vi "Socket.UDP Multicast Server.vi"() -> ()   [LabVIEW 2014]
uses:
  Classes/Socket.UDP/Socket.UDP.lvclass
  Classes/Socket.UDP/Socket.UDP.lvclass/Socket.UDP.ctl
  Classes/Socket.UDP/Accessors/Write time-to-live.vi
  Classes/Socket.UDP/Accessors/Write transfer_mode.vi
panel:
  out "error out":errorcluster
  in  "Stop Button":bool
  out "Transmitted Strings":string
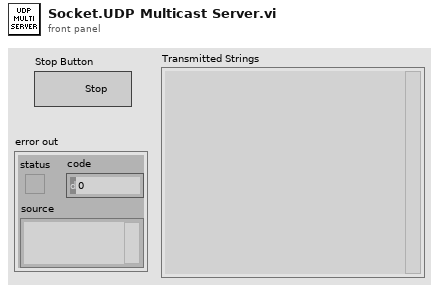
[diagram p1: front panel]
types:
  T1 = enum16{"point-to-point", "multicast", "broadcast"}
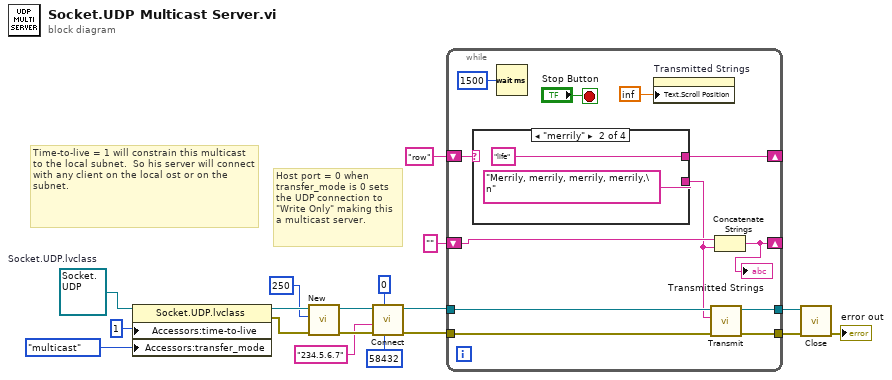
[diagram p0: block diagram]
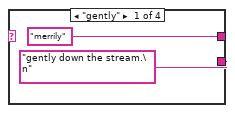
[diagram p2: hidden frame]
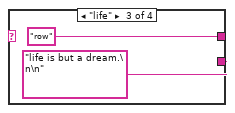
[diagram p3: hidden frame]
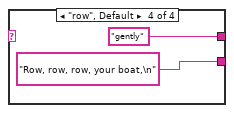
[diagram p4: hidden frame]
diagram:
  w18 = refnum<class "Socket.UDP.lvclass"> refnum  # Socket.UDP.lvclass
  # "Host port = 0 when transfer_mode is 0 sets  the UDP connection to \"Write Only\" making this a multicast server."
  # "Time-to-live = 1 will constrain this multicast to the local subnet.  So his server will connect with any client on the local ost or on the subnet."
  n1 = property class="Socket.UDP.lvclass"(reference=w18, "Accessors:time-to-live"=u16 1 ("time-to-live"), "Accessors:transfer_mode"=T1."multicast" ("transfer_mode")) -> (reference out=w17:refnum<class "Socket.UDP.lvclass">, error out=w15:errorcluster)  [unwired: 1 in]
  n2 = call-dynamic "New.vi"("error in (no error)"=w15, "timeout"=250, "Socket.UDP in"=w17) -> ("error out"=w11:errorcluster, "Socket.UDP out"=w12:refnum<class "Socket.UDP.lvclass">)  [unwired: 7 in]
  n3 = call-dynamic "Connect.vi"("remote_port"=u16 58432, "host_port"=u16 0, "error in (no error)"=w11, "remote_address"="234.5.6.7", "Socket.UDP in"=w12) -> ("error out"=w4:errorcluster, "Socket.UDP out"=w5:refnum<class "Socket.UDP.lvclass">)  [unwired: 5 in]
  n4 = while {
    shift-right: [w29] -> _
    shift-left: "row" -> [w30]
    shift-right: [w24] -> _
    shift-left: "" -> [w26]
    tunnel: w5 -> [w20]
    tunnel: w4 -> [w23]
    tunnel: [w21] -> w2
    tunnel: [w22] -> w3
    stop <- "Stop Button" stop-if-true
    n5 = case shown="\"merrily\"" w30 {
      tunnel: ["merrily" "life" "row" "gently"] -> w29
      tunnel: ["gently down the stream.\n" "Merrily, merrily, merrily, merrily,\n" "life is but a dream.\n\n" "Row, row, row, your boat,\n"] -> w19
      frame "gently" {
      }
      frame "merrily" {
      }
      frame "life" {
      }
      frame "row", Default {
      }
    }
    n6 = Wait (ms)(milliseconds to wait=u32 1500) -> ()  [unwired: 1 out]
    n7 = property on="Transmitted Strings" class="Str"("Text.Scroll Position"=inf) -> ()  [unwired: 2 in, 2 out]
    n8 = call-dynamic "Transmit.vi"("error in (no error)"=w23, "Data"=w19, "Socket.UDP in"=w20) -> ("error out"=w22:errorcluster, "Socket.UDP out"=w21:refnum<class "Socket.UDP.lvclass">)  [unwired: 6 in, 1 out]
    n9 = Concatenate Strings(w26, w19) -> (w24:string)
    "Transmitted Strings" <- w24
  }
  n10 = call-dynamic "Close.vi"("error in (no error)"=w3, "Socket.UDP in"=w2) -> ("error out"=→"error out":errorcluster)  [unwired: 8 in, 1 out]
